vi "PathToUNIXPathString.vi"(2 "error in (no error)":errorcluster, 3 "LV Path":path) -> (0 "error out":errorcluster, 1 "UNIX Path":string)   [LabVIEW 2017]
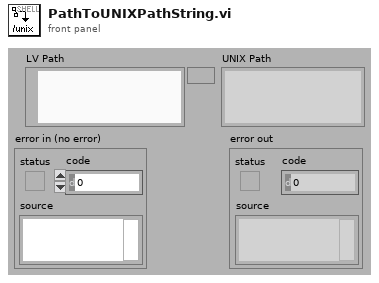
[diagram p1: front panel]
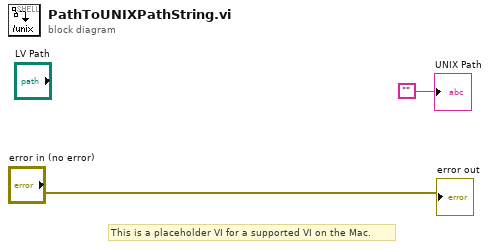
[diagram p0: block diagram]
diagram:
  # "This is a placeholder VI for a supported VI on the Mac."
  "error out" <- "error in (no error)"
  "UNIX Path" <- ""
